vi "Get Parameters from Hardware.vi"(8 "error in (no error)":errorcluster, 10 "Initial parameters":refnum<class "Mag Lab Parameters.lvclass">, 11 "Mag Lab Measure Base in":refnum<class "Mag Lab Measure Base.lvclass">) -> (0 "error out":errorcluster, 2 "Updated parameters":refnum<class "Mag Lab Parameters.lvclass">, 3 "Mag Lab Measure Base out":refnum<class "Mag Lab Measure Base.lvclass">)   [LabVIEW 2015, in "Mag Lab Measure Base.lvclass"]
uses:
  Mag Lab Measure Base.lvclass
  Mag Lab Properties/Mag Lab Parameters.lvclass
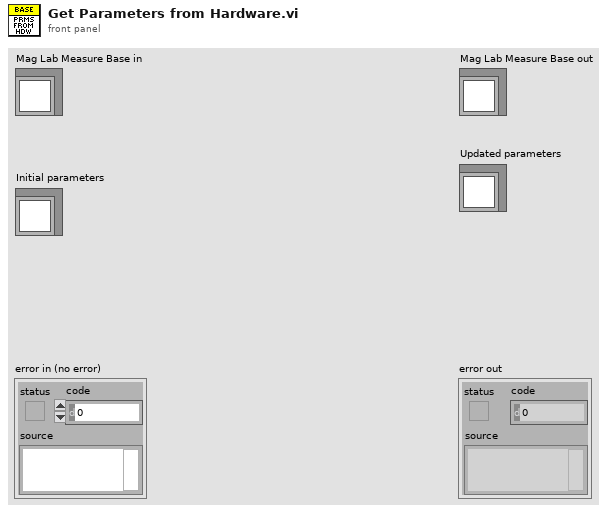
[diagram p1: front panel]
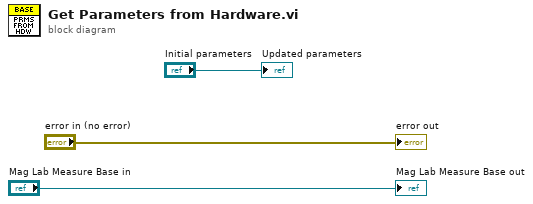
[diagram p0: block diagram]
diagram:
  "error out" <- "error in (no error)"
  "Mag Lab Measure Base out" <- "Mag Lab Measure Base in"
  "Updated parameters" <- "Initial parameters"
